vi "Open Py WND.vi"(8 "error in (no error)":errorcluster, 11 "Document Path":path) -> (0 "error out":errorcluster)   [LabVIEW 2019, in "Py Doc.lvclass"]
uses:
  Py Doc.lvclass
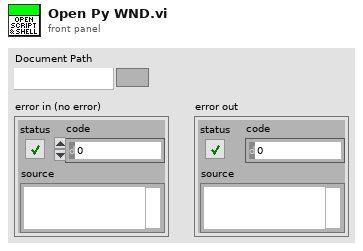
[diagram p1: front panel]
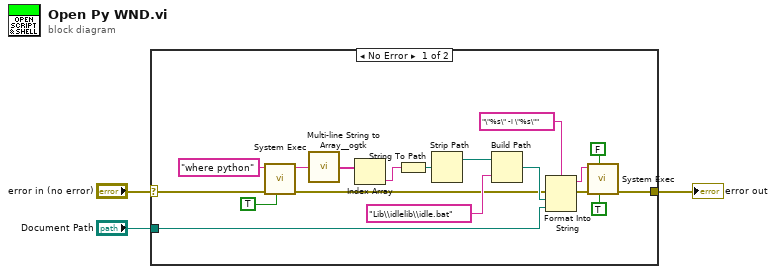
[diagram p0: block diagram]
diagram:
  n1 = case shown="No Error" "error in (no error)" {
    selector: "error in (no error)" -> [w19 w22]
    tunnel: "Document Path" -> [w21 _]
    tunnel: [w20 w22] -> w2
    frame No Error {
      n2 = call <vilib>:"System Exec.vi"("run minimized? (F)"=TRUE, "error in (no error)"=w19, "command line"="where python") -> ("error out"=w4:errorcluster, "standard output"=w16:string)  [unwired: 5 in, 2 out]
      n3 = call <userlib>:"Multi-line String to Array__ogtk.vi"("string"=w16) -> ("lines"=w15:string[])
      n4 = Index Array(array=w15) -> (element=w17:string)  [unwired: 1 in]
      n5 = String To Path(string=w17) -> (path=w8:path)
      n6 = Strip Path(path=w8) -> (stripped path=w7:path)  [unwired: 1 out]
      n7 = Build Path(base path=w7, name or relative path="Lib\\idlelib\\idle.bat") -> (appended path=w5:path)
      n8 = Format Into String(format string="\"%s\" -i \"%s\"", error in=w4, w5, w21) -> (resulting string=w13:string, error out=w14:errorcluster)  [unwired: 1 in]
      n9 = call <vilib>:"System Exec.vi"("run minimized? (F)"=TRUE, "wait until completion? (T)"=FALSE, "error in (no error)"=w14, "command line"=w13) -> ("error out"=w20:errorcluster)  [unwired: 4 in, 3 out]
    }
    frame Error {
    }
  }
  "error out" <- w2
